vi "Has Content.vi"(8 "Error In":errorcluster, 11 "Parser In":refnum<class "Parser.lvclass">) -> (0 "Error Out":errorcluster, 2 "Content":bool, 3 "Parser Out":refnum<class "Parser.lvclass">)   [LabVIEW 2017, in "Mustache.lvlib" / "Parser.lvclass"]
uses:
  Parser.lvclass
  Parser.lvclass/Parser.ctl
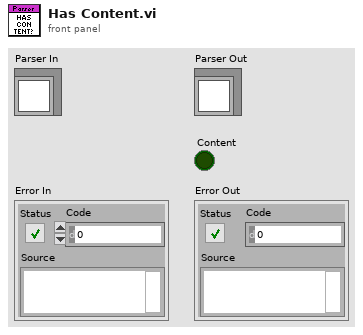
[diagram p1: front panel]
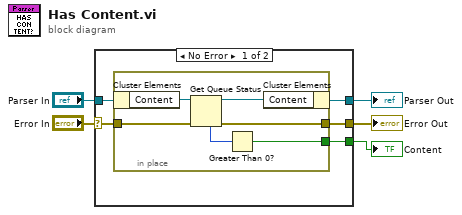
[diagram p0: block diagram]
diagram:
  n1 = case shown="No Error" "Error In" {
    selector: "Error In" -> [w7 w17]
    tunnel: [w10 w17] -> w5
    tunnel: "Parser In" -> [w9 w18]
    tunnel: [w8 w18] -> w3
    tunnel: [w6 _] -> w1
    frame No Error {
      n2 = in-place {
        in-place-border: w7 -> [w16]
        in-place-border: [w12] -> w10
        in-place-border: [w11] -> w6
        n3 = in-place-cluster #1(w9) -> ("Content"=w14:refnum<queue>)
        n4 = Get Queue Status(queue=w14, error in (no error)=w16) -> (queue out=w13:refnum<queue>, error out=w12:errorcluster, # elements in queue=w15:i32)  [unwired: 1 in, 5 out]
        n5 = Greater Than 0?(x=w15) -> (x > 0?=w11:bool)
        n6 = in-place-cluster #1("Content"=w13) -> (w8:refnum<class "Parser.lvclass">)
      }
    }
    frame Error {
    }
  }
  "Error Out" <- w5
  "Parser Out" <- w3
  "Content" <- w1
